vi "Copy.vi"(8 "error in (no error)":errorcluster, 10 "source in":refnum<class "NT Base.lvclass">, 11 "NT Scalar (Numeric) in":refnum<class "NT Scalar (Numeric).lvclass">) -> (0 "error out":errorcluster, 3 "NT Scalar (Numeric) out":refnum<class "NT Scalar (Numeric).lvclass">)   [LabVIEW 2020, in "PV Access.lvlib" / "PV Data.lvlib" / "NT Scalar (Numeric).lvclass"]
uses:
  NT Scalar (Numeric).lvclass
  NT Base/NT Base.lvclass
  NT Scalar (Numeric).lvclass/NT Scalar (Numeric).ctl
  NT Scalar/NT Scalar.lvclass
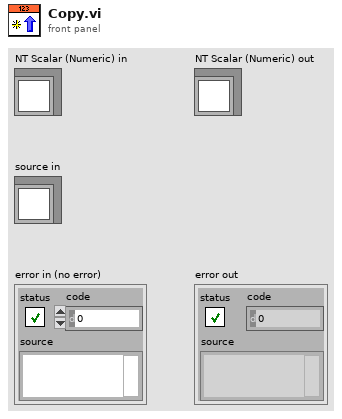
[diagram p1: front panel]
types:
  T1 = typedef "PV Access.lvlib/PV Data.lvlib/Alarm Limits.ctl" = cluster{"Active":bool, "Low Alarm Limit":variant, "Low Warning Limit":variant, "High Warning Limit":variant, "High Alarm Limit":variant, "Low Alarm Severity":T2, "Low Warning Severity":T2, "High Warning Severity ":T2, "High Alarm Severity":T2, "Hysteresis":dbl}
  T2 = typedef "PV Access.lvlib/PV Data.lvlib/Alarm Severity.ctl" = enum32{"no", "minor", "major", "record", "invalid", "undefined", ""}
  T3 = typedef "PV Access.lvlib/PV Data.lvlib/Control Metadata.ctl" = cluster{"Limit Low":variant, "Limit High":variant, "Min Step":variant}
  T4 = typedef "PV Access.lvlib/PV Data.lvlib/Display Form.ctl" = enum32{"Default", "String", "Binary", "Decimal", "Hex", "Exponential", "Engineering"}
  T5 = cluster{"Limit Low":variant, "Limit High":variant, "Units":string, "Precision":i32, "Form":T4}
  T6 = typedef "PV Access.lvlib/PV Data.lvlib/Value Fields.ctl" = cluster{"Display":bool, "Control":bool, "Alarm Limits":bool}
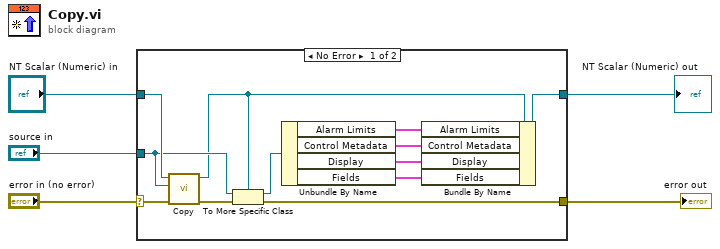
[diagram p0: block diagram]
diagram:
  n1 = case shown="No Error" "error in (no error)" {
    selector: "error in (no error)" -> [w17 w18]
    tunnel: [w9 w18] -> w5
    tunnel: [w11 w19] -> w4
    tunnel: "source in" -> [w8 _]
    tunnel: "NT Scalar (Numeric) in" -> [w16 w19]
    frame No Error {
      n2 = call-parent "Copy.vi"("error in (no error)"=w17, 10:"NT Base in"=w8, 11:"NT Base in"=w16) -> ("error out"=w10:errorcluster, "NT Base out"=w7:refnum<class "NT Scalar (Numeric).lvclass">)  [unwired: 7 in]
      n3 = To More Specific Class(target class=w7, reference=w8, error in=w10) -> (specific class reference=w6:refnum<class "NT Scalar (Numeric).lvclass">, error out=w9:errorcluster)
      n4 = Unbundle By Name(w6) -> ("Alarm Limits"=w15:T1, "Control Metadata"=w12:T3, "Display"=w13:T5, "Fields"=w14:T6)
      n5 = Bundle By Name(cluster=w7, "Alarm Limits"=w15, "Control Metadata"=w12, "Display"=w13, "Fields"=w14) -> (w11:refnum<class "NT Scalar (Numeric).lvclass">)
    }
    frame Error {
    }
  }
  "error out" <- w5
  "NT Scalar (Numeric) out" <- w4
